vi "Read Signature Fields.vi"(8 "error in (no error)":errorcluster, 11 "Session in":refnum<class "Session.lvclass">) -> (0 "error out":errorcluster, 2 "Signature Fields":T1, 3 "Session out":refnum<class "Session.lvclass">)   [LabVIEW 2015, in "NI_Azure_Core.lvlib" / "Session.lvclass"]
uses:
  Session.lvclass
  Signature Fields.ctl
  Session.lvclass/Session.ctl
  NI_Azure_Core.lvlib
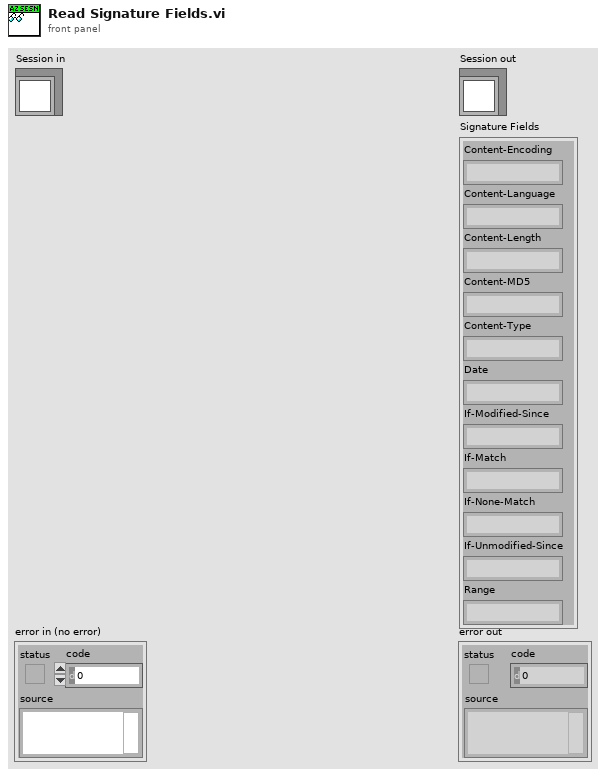
[diagram p1: front panel]
types:
  T1 = typedef "NI_Azure_Core.lvlib/Signature Fields.ctl" = cluster{"Content-Encoding":string, "Content-Language":string, "Content-Length":string, "Content-MD5":string, "Content-Type":string, "Date":string, "If-Modified-Since":string, "If-Match":string, "If-None-Match":string, "If-Unmodified-Since":string, "Range":string}
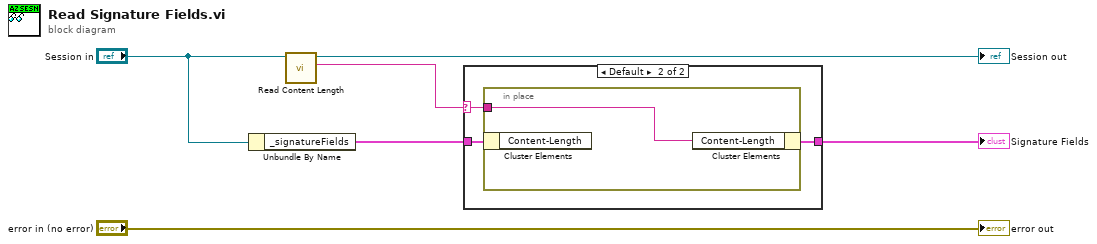
[diagram p0: block diagram]
diagram:
  n1 = Unbundle By Name("Session in") -> ("_signatureFields"=w5:T1)
  n2 = call "Read Content Length.vi"("Azure Session in"="Session in") -> ("Content length"=w1:string, "Azure Session out"=→"Session out":refnum<class "Session.lvclass">)  [unwired: 8 in, 1 out]
  n3 = case shown="Default" w1 {
    selector: w1 -> [_ w8]
    tunnel: w5 -> [w7 w10]
    tunnel: [w7 w9] -> w4
    frame "0" {
    }
    frame Default {
      n4 = in-place {
        in-place-border: w8 -> [w11]
        n5 = in-place-cluster #1(w10) -> ()  [unwired: 1 out]
        n6 = in-place-cluster #1("Content-Length"=w11) -> (w9:T1)
      }
    }
  }
  "Signature Fields" <- w4
  "error out" <- "error in (no error)"
